vi "Send command (standalone).vi"(3 "Value":u16, 4 "Command":T2=17 items=["Measured main TEC temperature"=0, "Measured SHG heater temperature"=1, "Measured BRF heater temperature"=2, "Main TEC temperature command"=3, "SHG heater temperature command"=4, "BRF heater temperature command"=5, "Main TEC drive"=6, "SHG heater drive"=7, "BRF heater drive"=8, "Output power from photodiode"=9, "Output power setpoint (Get)"=10, "Output power setpoint (Set)"=11, "Start-up power setting (Get)"=12, "Start-up power setting (Set)"=13, "Measured LDD current"=14, "Maximum LDD current limit"=15, "16-bit fault code"=16, "Head serial number"=17, "Head board rev"=18, "Head type"=19, "LDD enable state"=20, "Key switch command (Get)"=24, "Key switch command (Set)"=25, "Key switch actual"=26, "Interlock status"=27, "Head hours"=28, "Photo or current mode command (Get)"=29, "Photo or current mode command (Set)"=30, "Photo or current mode actual"=31, "Analog input enable command (Get)"=32, "Analog input enable command (Set)"=33, "Analog input actual"=34, "Power supply glue input"=36, "Power supply glue output"=37], 5 "Selected laser":T1 items=["Green Laser", "Blue Laser"]) -> (0 "Error":errorcluster, 1 "response value":sgl, 2 "response":string)   [LabVIEW 2018]
uses:
  Commands.ctl
  Laser enum.ctl
  Coherent global.vi
panel:
  # "PN 06/11/2014,\n      08/04/2019"
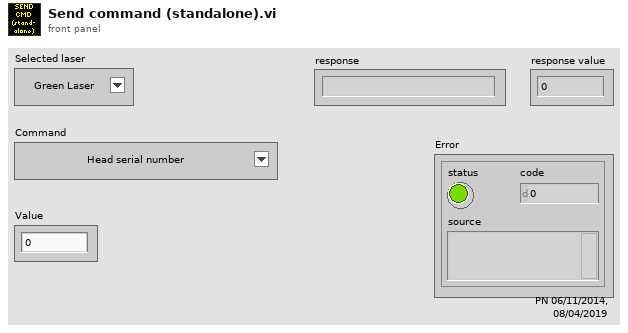
[diagram p1: front panel]
types:
  T1 = typedef "Laser enum.ctl" = u8
  T2 = typedef "Commands.ctl" = u8
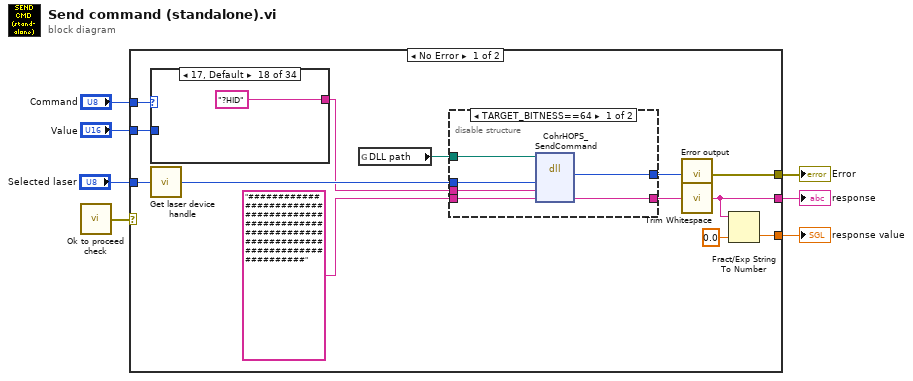
[diagram p0: block diagram]
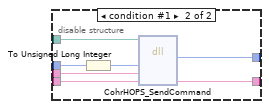
[diagram p2: hidden frame]
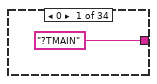
[diagram p3: hidden frame]
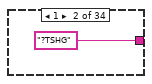
[diagram p4: hidden frame]
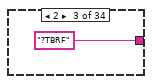
[diagram p5: hidden frame]
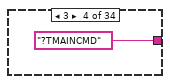
[diagram p6: hidden frame]
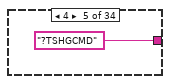
[diagram p7: hidden frame]
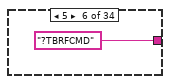
[diagram p8: hidden frame]
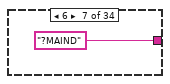
[diagram p9: hidden frame]
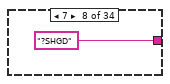
[diagram p10: hidden frame]
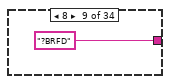
[diagram p11: hidden frame]
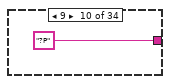
[diagram p12: hidden frame]
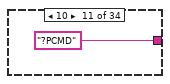
[diagram p13: hidden frame]
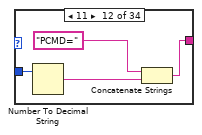
[diagram p14: hidden frame]
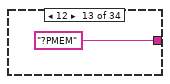
[diagram p15: hidden frame]
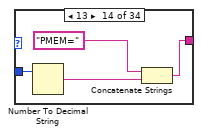
[diagram p16: hidden frame]
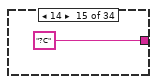
[diagram p17: hidden frame]
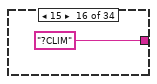
[diagram p18: hidden frame]
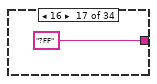
[diagram p19: hidden frame]
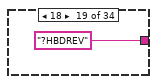
[diagram p20: hidden frame]
diagram:
  n1 = call "Ok to proceed check.vi"() -> ("Error"=w7:errorcluster)
  n2 = case shown="No Error" w7 {
    selector: w7 -> [_ w85]
    tunnel: [w19 sgl 0.0] -> w6
    tunnel: [w18 "" ("trimmed string")] -> w5
    tunnel: [w17 w85] -> w4
    tunnel: "Command" -> [w16 _]
    tunnel: "Value" -> [w15 _]
    tunnel: "Selected laser" -> [w14 _]
    frame No Error {
      n3 = case shown="17, Default" w16 {
        tunnel: ["?TMAIN" "?TSHG" "?TBRF" "?TMAINCMD" "?TSHGCMD" "?TBRFCMD" "?MAIND" "?SHGD" "?BRFD" "?P" "?PCMD" w45 "?PMEM" w50 "?C" "?CLIM" "?FF" "?HID" "?HBDREV" "?HTYPE" "?L" "?KSWCMD" w63 "?KSW" "?INT" "?HH" "?CMODECMD" w71 "?CMODE" "?ANACMD" w77 "?ANA" "?PSGLUEIN" "?PSGLUEOUT"] -> w11
        tunnel: w15 -> [_ _ _ _ _ _ _ _ _ _ _ w48 _ w53 _ _ _ _ _ _ _ _ w65 _ _ _ _ w73 _ _ w79 _ _ _]
        frame 0 {
        }
        frame 1 {
        }
        frame 2 {
        }
        frame 3 {
        }
        frame 4 {
        }
        frame 5 {
        }
        frame 6 {
        }
        frame 7 {
        }
        frame 8 {
        }
        frame 9 {
        }
        frame 10 {
        }
        frame 11 {
          n4 = Number To Decimal String(number=w48) -> (decimal integer string=w47:string)  [unwired: 1 in]
          n5 = Concatenate Strings("PCMD=", w47) -> (w45:string)
        }
        frame 12 {
        }
        frame 13 {
          n6 = Number To Decimal String(number=w53) -> (decimal integer string=w52:string)  [unwired: 1 in]
          n7 = Concatenate Strings("PMEM=", w52) -> (w50:string)
        }
        frame 14 {
        }
        frame 15 {
        }
        frame 16 {
        }
        frame 17, Default {
        }
        frame 18 {
        }
        frame 19 {
        }
        frame 20 {
        }
        frame 24 {
        }
        frame 25 {
          n8 = Number To Decimal String(number=w65) -> (decimal integer string=w62:string)  [unwired: 1 in]
          n9 = Concatenate Strings("KSWCMD=", w62) -> (w63:string)
        }
        frame 26 {
        }
        frame 27 {
        }
        frame 28 {
        }
        frame 29 {
        }
        frame 30 {
          n10 = Number To Decimal String(number=w73) -> (decimal integer string=w70:string)  [unwired: 1 in]
          n11 = Concatenate Strings("CMODECMD=", w70) -> (w71:string)
        }
        frame 31 {
        }
        frame 32 {
        }
        frame 33 {
          n12 = Number To Decimal String(number=w79) -> (decimal integer string=w76:string)  [unwired: 1 in]
          n13 = Concatenate Strings("ANACMD=", w76) -> (w77:string)
        }
        frame 34 {
        }
        frame 36 {
        }
        frame 37 {
        }
      }
      n14 = call "Get laser device handle.vi"("Selected laser"=w14) -> ("Device handle"=w12:u64)
      n15 = global read "Coherent global.vi" "DLL path"() -> (w13:path)
      n16 = disable-structure shown="TARGET_BITNESS==64" {
        disable-tunnel: "####################################################################################################" ("headType") -> [w26 w30]
        disable-tunnel: w11 -> [w25 w31]
        disable-tunnel: [w24 w28] -> w9
        disable-tunnel: [w23 w29] -> w8
        disable-tunnel: w12 -> [w22 w32]
        disable-tunnel: w13 -> [w21 w33]
        frame condition #0 (active) {
          n17 = dll-call lib="?" fn="CohrHOPS_SendCommand"(path in=w21, "handle"=w22, "command"=w25, "response"=w26) -> ("return value"=w24:i32, "response"=w23:string)  [unwired: 4 in, 2 out]
        }
        frame condition #1 {
          n18 = To Unsigned Long Integer(number=w32) -> (unsigned 32bit integer=w27:u32)
          n19 = dll-call lib="?" fn="CohrHOPS_SendCommand"(path in=w33, "handle"=w27, "command"=w31, "response"=w30) -> ("return value"=w28:i32, "response"=w29:string)  [unwired: 4 in, 2 out]
        }
      }
      n20 = call "Error output.vi"("I32 err code"=w9) -> ("Error Out"=w17:errorcluster)
      n21 = call <vilib>:"Trim Whitespace.vi"("string"=w8) -> ("trimmed string"=w18:string)  [unwired: 1 in]
      n22 = Fract/Exp String To Number(string=w18, default (0 dbl)=sgl 0.0 ("default (0 DBL)")) -> (number=w19:sgl)  [unwired: 2 in, 1 out]
    }
    frame Error {
    }
  }
  "response" <- w5
  "response value" <- w6
  "Error" <- w4
